vi "AudioFileCompleteBroadcast_Send.vi"(8 "error in (no error)":errorcluster, 9 "Audio File Complete":T1, 11 "Qbus":refnum<class "Qbus.lvclass">) -> (0 "error out":errorcluster, 3 "Qbus out":refnum<class "Qbus.lvclass">)   [LabVIEW 2017, in "EmsaAudio.lvlib"]
uses:
  <vilib>/addons/InsightCM/Devices/Shared/Emsa/EmsaAudio/EmsaAudio.lvlib
  <vilib>/addons/Qbus/Qbus.lvclass
  <vilib>/addons/InsightCM/Devices/Shared/Emsa/EmsaAudio/controls/AudioFileCompleteBroadcast.ctl
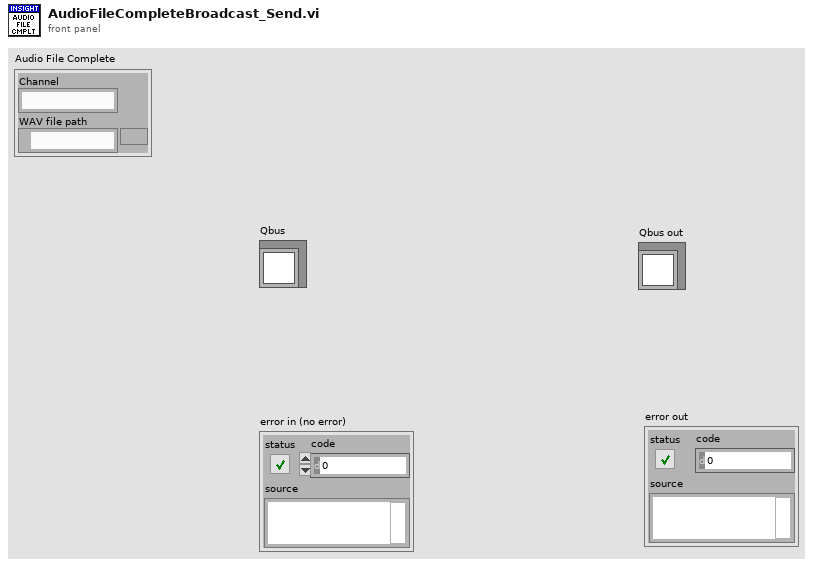
[diagram p1: front panel]
types:
  T1 = typedef "EmsaAudio.lvlib/AudioFileCompleteBroadcast.ctl" = cluster{"Channel":string, "WAV file path":path}
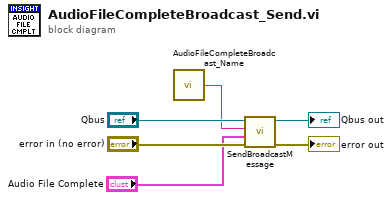
[diagram p0: block diagram]
diagram:
  n1 = call <vilib>:"AudioFileCompleteBroadcast_Name.vi"() -> ("message name"=w2:string)  [unwired: 5 in]
  n2 = call <vilib>:"SendBroadcastMessage.vi"("error in (no error)"="error in (no error)", "message value"="Audio File Complete", "message name"=w2, "Qbus in"="Qbus") -> ("error in (no error)"=→"error out":errorcluster, "Qbus out"=→"Qbus out":refnum<class "Qbus.lvclass">)  [unwired: 6 in]
